vi "Read Solution.vi"(8 "error in (no error)":errorcluster, 11 "Module Data in":refnum<class "Grassfire Algorithm.lvclass">) -> (0 "error out":errorcluster, 2 "Solution":T1[][](array[typedef]), 3 "Module Data out":refnum<class "Grassfire Algorithm.lvclass">)   [LabVIEW 2019, in "Grassfire Algorithm.lvclass"]
uses:
  Grassfire Algorithm.lvclass
  Solution Grid Cell--cluster.ctl
  Solution--picture ring.ctl
  Grassfire Algorithm.lvclass/Grassfire Algorithm.ctl
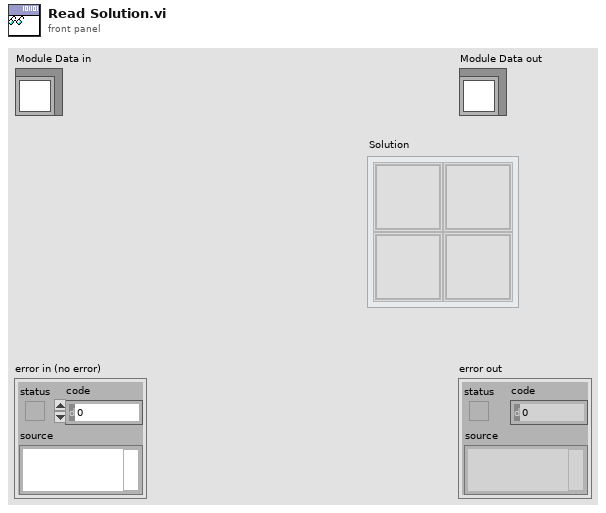
[diagram p1: front panel]
types:
  T1 = typedef "Grassfire Algorithm.lvclass/Solution Grid Cell--cluster.ctl" = cluster{"Picture":T2, "Value":string}
  T2 = typedef "Grassfire Algorithm.lvclass/Solution--picture ring.ctl" = i64
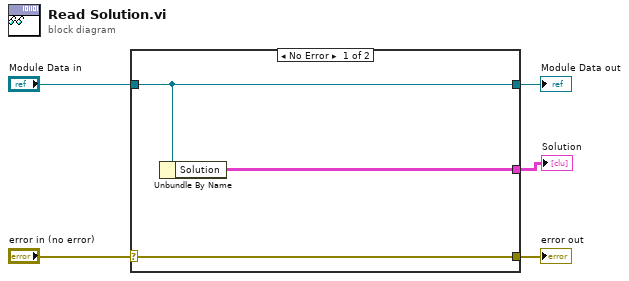
[diagram p0: block diagram]
diagram:
  n1 = case shown="No Error" "error in (no error)" {
    selector: "error in (no error)" -> [w8 w9]
    tunnel: [w8 w9] -> w4
    tunnel: [w7 w10] -> w2
    tunnel: "Module Data in" -> [w7 w10]
    tunnel: [w6 _] -> w1
    frame No Error {
      n2 = Unbundle By Name(w7) -> ("Solution"=w6:T1[][])
    }
    frame Error {
    }
  }
  "error out" <- w4
  "Module Data out" <- w2
  "Solution" <- w1
